vi "return zero.vi"(7 "Axis":enum16{"X", "Y", "X+Y"}(ring), 8 "error IN":errorcluster, 11 "Data IN":T1={"App State"="", "Connect "=FALSE, "phandle out"=0, "Axis"=[], "S ramp"=30.0, "Acceleration"=100000.0, "Initial Speed"=10.0, "Normal Open / Close"=enum."Close", "Deceleration"=100000.0, "Creep"=30.0, "Speed"=1000.0, "X Axis"={"Operating State"="", "Current Position"=0.0, "Current Speed"=0.0, "Axis State"=0, "Angle"=0.0}, "Y Axis"={"Operating State"="", "Current Position"=0.0, "Current Speed"=0.0, "Axis State"=0, "Angle"=0.0}, "Distance"=0.0, "Direct of movement"=enum."Forward", "Move Method"=enum."Continue", "Move Mode"=enum."Relative", "Angle"=enum."0", "Times"=0, "Start Time"=0.0, "Step Flag"=FALSE, "x  dist"=[], "y dist"=[], "x angle array"=[], "y angle array"=[], "index"=0.0, "big motion angle"=0.0, "big angle"=[], "xy dy speed table"=[], "x dy speed table"=[], "y dy speed table"=[], "x dy time"=[], "y dy time"=[], "xy dy time"=[], "dy Path  "=[]}) -> (0 "error out":errorcluster, 3 "Data out":T1={"App State"="", "Connect "=FALSE, "phandle out"=0, "Axis"=[], "S ramp"=30.0, "Acceleration"=100000.0, "Initial Speed"=10.0, "Normal Open / Close"=enum."Close", "Deceleration"=100000.0, "Creep"=30.0, "Speed"=1000.0, "X Axis"={"Operating State"="", "Current Position"=0.0, "Current Speed"=0.0, "Axis State"=0, "Angle"=0.0}, "Y Axis"={"Operating State"="", "Current Position"=0.0, "Current Speed"=0.0, "Axis State"=0, "Angle"=0.0}, "Distance"=0.0, "Direct of movement"=enum."Forward", "Move Method"=enum."Continue", "Move Mode"=enum."Relative", "Angle"=enum."0", "Times"=0, "Start Time"=0.0, "Step Flag"=FALSE, "x  dist"=[], "y dist"=[], "x angle array"=[], "y angle array"=[], "index"=0.0, "big motion angle"=0.0, "big angle"=[], "xy dy speed table"=[], "x dy speed table"=[], "y dy speed table"=[], "x dy time"=[], "y dy time"=[], "xy dy time"=[], "dy Path  "=[]})   [LabVIEW 2015]
uses:
  Typedef/Data2.ctl
  zauxdll-2014/zauxdll.lvlib
panel:
  # "m"
  # "m"
  # "m"
  # "m"
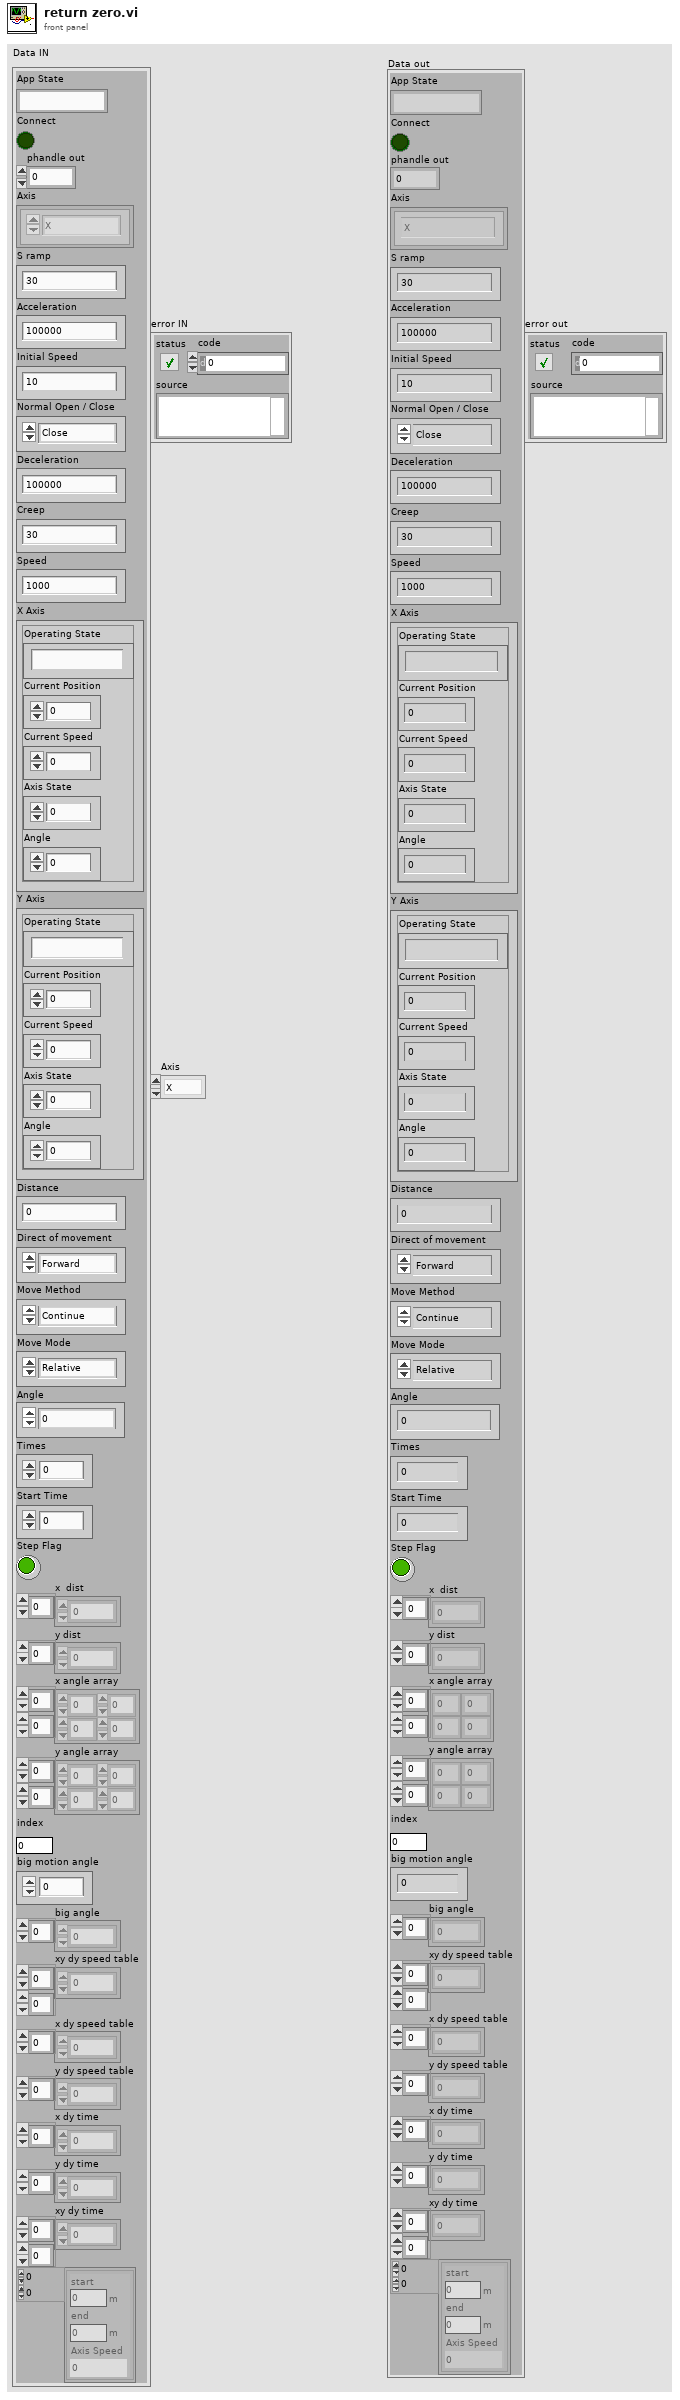
[diagram p1: front panel]
types:
  T1 = typedef "Data2.ctl" = cluster{"App State":string, "Connect ":bool, "phandle out":u32, "Axis":enum16{"X", "Y", "X+Y"}[], "S ramp":dbl, "Acceleration":dbl, "Initial Speed":dbl, "Normal Open / Close":enum16{"Open", "Close"}, "Deceleration":dbl, "Creep":dbl, "Speed":dbl, "X Axis":cluster{"Operating State":string, "Current Position":dbl, "Current Speed":dbl, "Axis State":i32, "Angle":dbl}, "Y Axis":cluster{"Operating State":string, "Current Position":dbl, "Current Speed":dbl, "Axis State":i32, "Angle":dbl}, "Distance":dbl, "Direct of movement":enum16{"Forward", "Backward"}, "Move Method":enum16{"Continue", "Inching"}, "Move Mode":enum16{"Relative", "Absolute"}, "Angle":enum32{"0", "1", "10", "30", "34", "60", "90", "180", "-1", "-10"}, "Times":i32, "Start Time":dbl, "Step Flag":bool, "x  dist":dbl[], "y dist":dbl[], "x angle array":i32[][], "y angle array":i32[][], "index":dbl, "big motion angle":dbl, "big angle":dbl[], "xy dy speed table":dbl[][], "x dy speed table":dbl[], "y dy speed table":dbl[], "x dy time":dbl[], "y dy time":dbl[], "xy dy time":dbl[][], "dy Path  ":cluster{"end":dbl, "start":dbl, "Axis Speed":dbl}[][]}
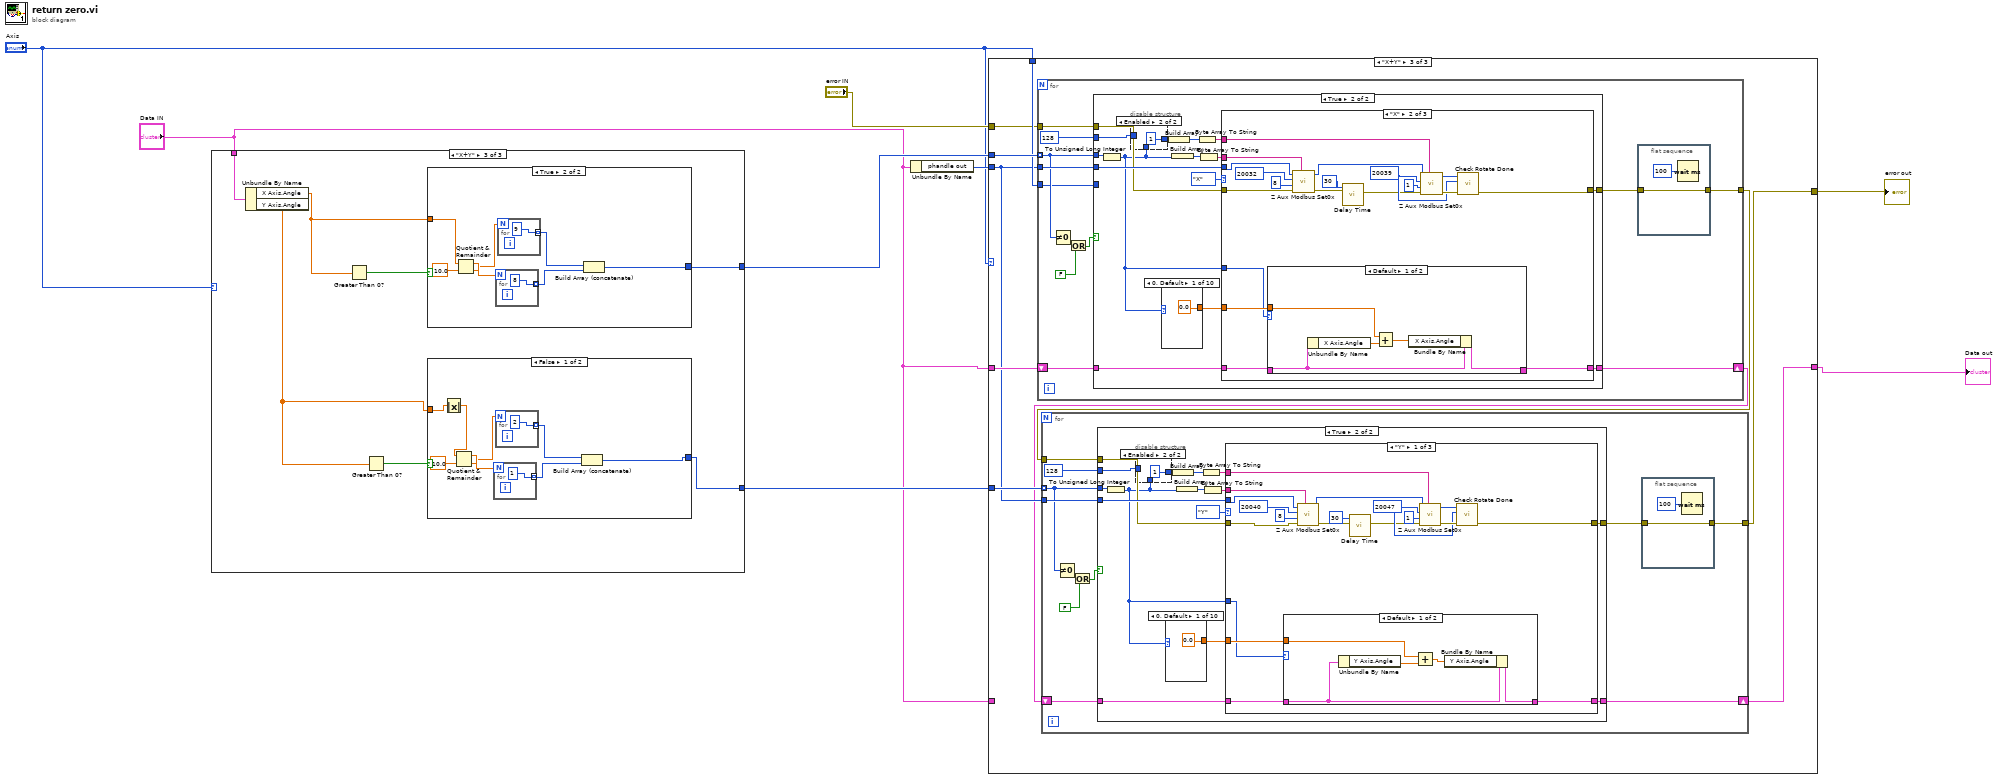
[diagram p0: block diagram]
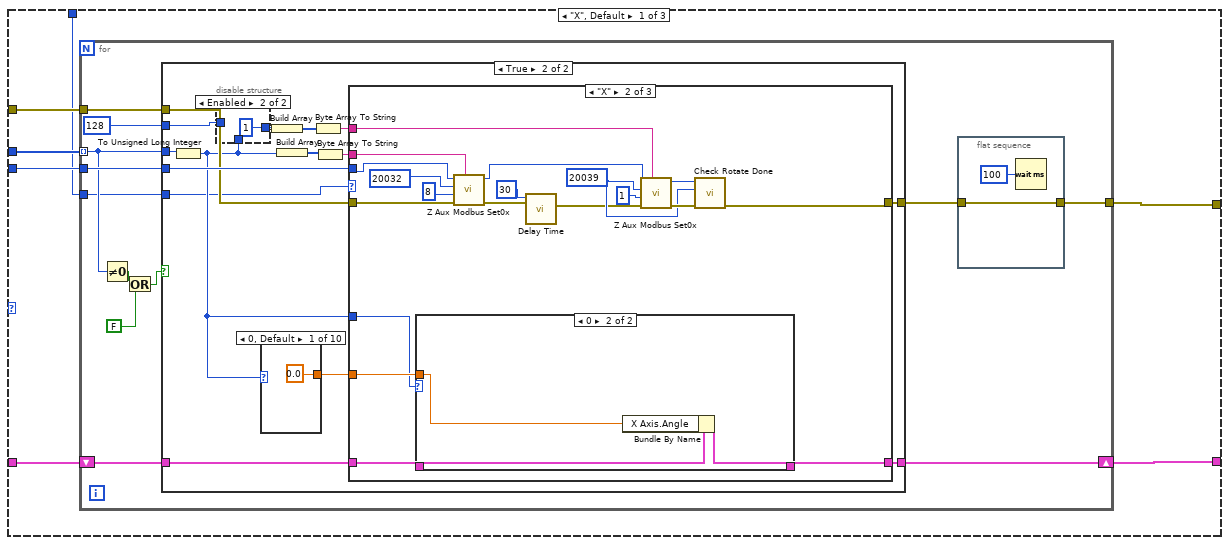
[diagram p2: hidden frame]
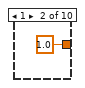
[diagram p4: hidden frame]
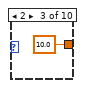
[diagram p5: hidden frame]
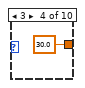
[diagram p6: hidden frame]
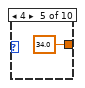
[diagram p7: hidden frame]
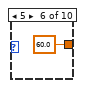
[diagram p8: hidden frame]
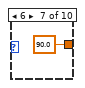
[diagram p9: hidden frame]
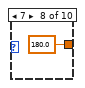
[diagram p10: hidden frame]
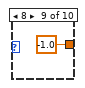
[diagram p11: hidden frame]
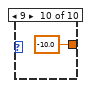
[diagram p12: hidden frame]
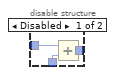
[diagram p13: hidden frame]
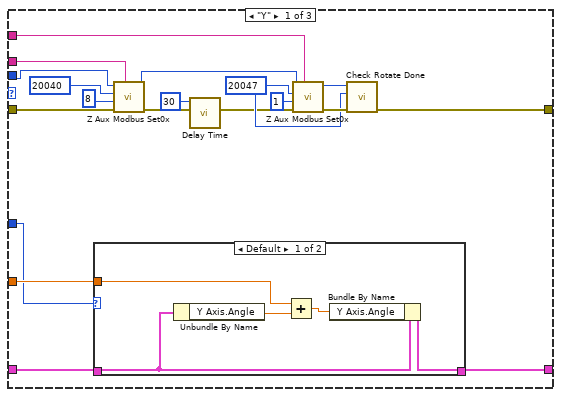
[diagram p14: hidden frame]
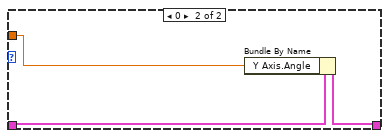
[diagram p15: hidden frame]
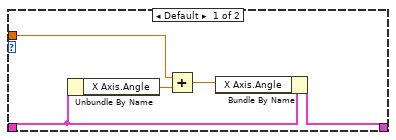
[diagram p16: hidden frame]
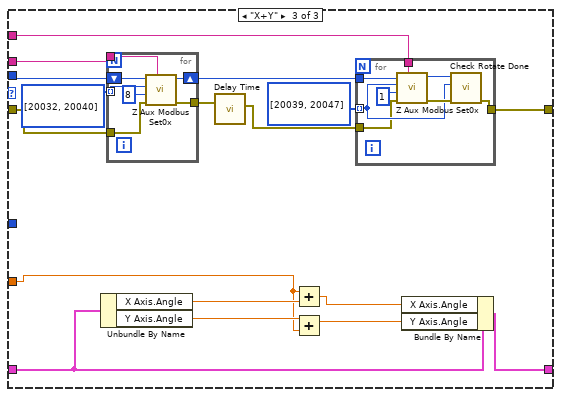
[diagram p17: hidden frame]
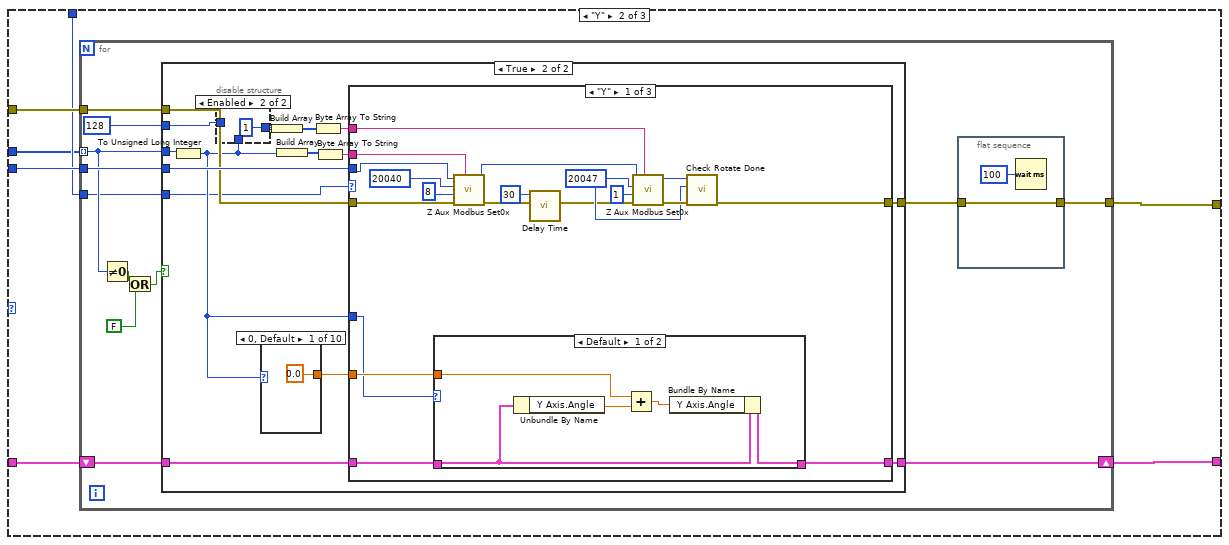
[diagram p18: hidden frame]
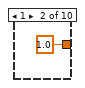
[diagram p20: hidden frame]
diagram:
  n1 = case shown="\"X+Y\"" "Axis" {
    tunnel: "Data IN" -> [w12 w35 w61]
    tunnel: [w9 w32 w58] -> w6
    tunnel: [_ _ w55] -> w4
    frame "X", Default {
      n2 = Unbundle By Name(w12) -> ("X Axis.Angle"=w10:dbl)
      n3 = Greater Than 0?(x=w10) -> (x > 0?=w11:bool)
      n4 = case shown="True" w11 {
        tunnel: w10 -> [w14 w29]
        tunnel: [w15 w23] -> w9
        frame False {
          n5 = Absolute Value(x=w14) -> (abs(x)=w13:dbl)
          n6 = Quotient & Remainder(x=w13, y=10.0) -> (x-y*floor(x/y)=w19:dbl, floor(x/y)=w18:dbl)
          n7 = for {
            N: w19 -> [_]
            tunnel: [1] -> w16 mode=indexing
          }
          n8 = for {
            N: w18 -> [_]
            tunnel: [2] -> w17 mode=indexing
          }
          n9 = Build Array (concatenate)(w17, w16) -> (w15:i32[])
        }
        frame True {
          n10 = Quotient & Remainder(x=w29, y=10.0) -> (x-y*floor(x/y)=w27:dbl, floor(x/y)=w26:dbl)
          n11 = for {
            N: w27 -> [_]
            tunnel: [8] -> w24 mode=indexing
          }
          n12 = for {
            N: w26 -> [_]
            tunnel: [9] -> w25 mode=indexing
          }
          n13 = Build Array (concatenate)(w25, w24) -> (w23:i32[])
        }
      }
    }
    frame "Y" {
      n14 = Unbundle By Name(w35) -> ("Y Axis.Angle"=w33:dbl)
      n15 = Greater Than 0?(x=w33) -> (x > 0?=w34:bool)
      n16 = case shown="True" w34 {
        tunnel: w33 -> [w37 w52]
        tunnel: [w38 w46] -> w32
        frame False {
          n17 = Absolute Value(x=w37) -> (abs(x)=w36:dbl)
          n18 = Quotient & Remainder(x=w36, y=10.0) -> (x-y*floor(x/y)=w42:dbl, floor(x/y)=w41:dbl)
          n19 = for {
            N: w42 -> [_]
            tunnel: [1] -> w39 mode=indexing
          }
          n20 = for {
            N: w41 -> [_]
            tunnel: [2] -> w40 mode=indexing
          }
          n21 = Build Array (concatenate)(w40, w39) -> (w38:i32[])
        }
        frame True {
          n22 = Quotient & Remainder(x=w52, y=10.0) -> (x-y*floor(x/y)=w50:dbl, floor(x/y)=w49:dbl)
          n23 = for {
            N: w50 -> [_]
            tunnel: [8] -> w47 mode=indexing
          }
          n24 = for {
            N: w49 -> [_]
            tunnel: [9] -> w48 mode=indexing
          }
          n25 = Build Array (concatenate)(w48, w47) -> (w46:i32[])
        }
      }
    }
    frame "X+Y" {
      n26 = Unbundle By Name(w61) -> ("X Axis.Angle"=w59:dbl, "Y Axis.Angle"=w56:dbl)
      n27 = Greater Than 0?(x=w59) -> (x > 0?=w60:bool)
      n28 = Greater Than 0?(x=w56) -> (x > 0?=w57:bool)
      n29 = case shown="True" w60 {
        tunnel: w59 -> [w82 w97]
        tunnel: [w83 w91] -> w58
        frame False {
          n30 = Absolute Value(x=w82) -> (abs(x)=w81:dbl)
          n31 = Quotient & Remainder(x=w81, y=10.0) -> (x-y*floor(x/y)=w87:dbl, floor(x/y)=w86:dbl)
          n32 = for {
            N: w87 -> [_]
            tunnel: [1] -> w84 mode=indexing
          }
          n33 = for {
            N: w86 -> [_]
            tunnel: [2] -> w85 mode=indexing
          }
          n34 = Build Array (concatenate)(w85, w84) -> (w83:i32[])
        }
        frame True {
          n35 = Quotient & Remainder(x=w97, y=10.0) -> (x-y*floor(x/y)=w95:dbl, floor(x/y)=w94:dbl)
          n36 = for {
            N: w95 -> [_]
            tunnel: [8] -> w92 mode=indexing
          }
          n37 = for {
            N: w94 -> [_]
            tunnel: [9] -> w93 mode=indexing
          }
          n38 = Build Array (concatenate)(w93, w92) -> (w91:i32[])
        }
      }
      n39 = case shown="False" w57 {
        tunnel: w56 -> [w63 w78]
        tunnel: [w64 w72] -> w55
        frame False {
          n40 = Absolute Value(x=w63) -> (abs(x)=w62:dbl)
          n41 = Quotient & Remainder(x=w62, y=10.0) -> (x-y*floor(x/y)=w68:dbl, floor(x/y)=w67:dbl)
          n42 = for {
            N: w68 -> [_]
            tunnel: [1] -> w65 mode=indexing
          }
          n43 = for {
            N: w67 -> [_]
            tunnel: [2] -> w66 mode=indexing
          }
          n44 = Build Array (concatenate)(w66, w65) -> (w64:i32[])
        }
        frame True {
          n45 = Quotient & Remainder(x=w78, y=10.0) -> (x-y*floor(x/y)=w76:dbl, floor(x/y)=w75:dbl)
          n46 = for {
            N: w76 -> [_]
            tunnel: [8] -> w73 mode=indexing
          }
          n47 = for {
            N: w75 -> [_]
            tunnel: [9] -> w74 mode=indexing
          }
          n48 = Build Array (concatenate)(w74, w73) -> (w72:i32[])
        }
      }
    }
  }
  n49 = Unbundle By Name("Data IN") -> ("phandle out"=w8:u32)
  n50 = case shown="\"X+Y\"" "Axis" {
    tunnel: w8 -> [w106 w244 w380]
    tunnel: "error IN" -> [w105 w243 w382]
    tunnel: "Data IN" -> [w104 w242 w385]
    tunnel: w6 -> [w103 w238 w384]
    tunnel: [w102 w241 w377] -> w1
    tunnel: "Axis" -> [w101 w240 w383]
    tunnel: w4 -> [_ _ w381]
    tunnel: "Data IN" -> [_ _ _]
    tunnel: [w100 w239 w378] -> w2
    frame "X", Default {
      n51 = for {
        tunnel: w106 -> [w114]
        tunnel: w105 -> [w118]
        tunnel: w103 -> [w113] mode=indexing
        shift-right: [w115] -> w102
        shift-left: w104 -> [w116]
        tunnel: [w109] -> w100
        tunnel: w101 -> [w107]
        n52 = Not Equal To 0?(x=w113) -> (x != 0?=w111:bool)
        n53 = Or(x=w111, y=FALSE) -> (x .or. y?=w112:bool)
        n54 = case shown="True" w112 {
          tunnel: w114 -> [_ w137]
          tunnel: w118 -> [w122 w136]
          tunnel: u32 128 -> [_ w135]
          tunnel: w116 -> [w121 w129]
          tunnel: w113 -> [_ w128]
          tunnel: [w121 w127] -> w115
          tunnel: [w122 w126] -> w110
          tunnel: w107 -> [_ w123]
          frame False {
          }
          frame True {
            n55 = To Unsigned Long Integer(number=w128) -> (unsigned 32bit integer=w124:u32)
            n56 = disable-structure shown="Enabled" {
              disable-tunnel: w135 -> [w150 _]
              disable-tunnel: [w149 u32 1] -> w134
              disable-tunnel: w124 -> [w148 _]
              frame Disabled {
                n57 = Add(x=w150, y=w148) -> (x+y=w149:u32)
              }
              frame Enabled {
              }
            }
            n58 = case shown="0, Default" w124 {
              tunnel: [0.0 1.0 10.0 30.0 34.0 60.0 90.0 180.0 -1.0 -10.0] -> w130
              frame 0, Default {
              }
              frame 1 {
              }
              frame 2 {
              }
              frame 3 {
              }
              frame 4 {
              }
              frame 5 {
              }
              frame 6 {
              }
              frame 7 {
              }
              frame 8 {
              }
              frame 9 {
              }
            }
            n59 = Build Array(w134) -> (w133:u32[])
            n60 = Build Array(w124) -> (w125:u32[])
            n61 = Byte Array To String(unsigned byte array=w133) -> (string=w132:string)
            n62 = Byte Array To String(unsigned byte array=w125) -> (string=w131:string)
            n63 = case shown="\"X\"" w123 {
              tunnel: w137 -> [w167 w194 w221]
              tunnel: w132 -> [w168 w195 w222]
              tunnel: w131 -> [w166 w193 w220]
              tunnel: w136 -> [w161 w188 w217]
              tunnel: [w156 w183 w213] -> w126
              tunnel: w129 -> [w155 w182 w210]
              tunnel: [w154 w181 w209] -> w127
              tunnel: w130 -> [w153 w180 w206]
              tunnel: w124 -> [w152 w179 _]
              frame "Y" {
                w162 = u16 20047 ("start")
                n64 = case shown="Default" w152 {
                  tunnel: w155 -> [w175 w178]
                  tunnel: [w174 w177] -> w154
                  tunnel: w153 -> [w171 w176]
                  frame Default {
                    n65 = Unbundle By Name(w175) -> ("Y Axis.Angle"=w172:dbl)
                    n66 = Add(x=w171, y=w172) -> (x+y=w173:dbl)
                    n67 = Bundle By Name(cluster=w175, "Y Axis.Angle"=w173) -> (w174:T1)
                  }
                  frame 0 {
                    n68 = Bundle By Name(cluster=w178, "Y Axis.Angle"=w176) -> (w177:T1)
                  }
                }
                n69 = call "Z Aux Modbus Set0x.vi"("pdata"=w166, "error in (no error)"=w161, "inum"=u16 8, "start"=u16 20040, "handle"=w167) -> ("error out"=w159:errorcluster, "handle out"=w160:u32)  [unwired: 3 in, 2 out]
                n70 = call "Delay Time.vi"("error in (no error)"=w159, "Delay(ms)"=u32 30) -> ("error out"=w157:errorcluster)  [unwired: 9 in]
                n71 = call "Z Aux Modbus Set0x.vi"("pdata"=w168, "error in (no error)"=w157, "inum"=u16 1, "start"=w162, "handle"=w160) -> ("error out"=w170:errorcluster, "handle out"=w169:u32)  [unwired: 3 in, 2 out]
                n72 = call "Check Rotate Done.vi"("error in (no error)"=w170, "start"=w162, "phandle in"=w169) -> ("error out"=w156:errorcluster)  [unwired: 8 in]
              }
              frame "X" {
                w189 = u16 20039 ("start")
                n73 = case shown="0" w179 {
                  tunnel: w182 -> [w202 w205]
                  tunnel: [w201 w204] -> w181
                  tunnel: w180 -> [w198 w203]
                  frame Default {
                    n74 = Unbundle By Name(w202) -> ("X Axis.Angle"=w200:dbl)
                    n75 = Add(x=w198, y=w200) -> (x+y=w199:dbl)
                    n76 = Bundle By Name(cluster=w202, "X Axis.Angle"=w199) -> (w201:T1)
                  }
                  frame 0 {
                    n77 = Bundle By Name(cluster=w205, "X Axis.Angle"=w203) -> (w204:T1)
                  }
                }
                n78 = call "Z Aux Modbus Set0x.vi"("pdata"=w193, "error in (no error)"=w188, "inum"=u16 8, "start"=u16 20032, "handle"=w194) -> ("error out"=w186:errorcluster, "handle out"=w187:u32)  [unwired: 3 in, 2 out]
                n79 = call "Delay Time.vi"("error in (no error)"=w186, "Delay(ms)"=u32 30) -> ("error out"=w184:errorcluster)  [unwired: 9 in]
                n80 = call "Z Aux Modbus Set0x.vi"("pdata"=w195, "error in (no error)"=w184, "inum"=u16 1, "start"=w189, "handle"=w187) -> ("error out"=w197:errorcluster, "handle out"=w196:u32)  [unwired: 3 in, 2 out]
                n81 = call "Check Rotate Done.vi"("error in (no error)"=w197, "start"=w189, "phandle in"=w196) -> ("error out"=w183:errorcluster)  [unwired: 8 in]
              }
              frame "X+Y" {
                n82 = Unbundle By Name(w210) -> ("X Axis.Angle"=w212:dbl, "Y Axis.Angle"=w211:dbl)
                n83 = for {
                  tunnel: w220 -> [w236]
                  shift-right: [w235] -> w215
                  shift-left: w221 -> [w237]
                  tunnel: i32[] [20032, 20040] -> [w233] mode=indexing
                  tunnel: w217 -> [w232]
                  tunnel: [w231] -> w216
                  n84 = call "Z Aux Modbus Set0x.vi"("pdata"=w236, "error in (no error)"=w232, "inum"=u16 8, "start"=w233, "handle"=w237) -> ("error out"=w231:errorcluster, "handle out"=w235:u32)  [unwired: 3 in, 2 out]
                }
                n85 = call "Delay Time.vi"("error in (no error)"=w216) -> ("error out"=w214:errorcluster)  [unwired: 10 in]
                n86 = Add(x=w206, y=w212) -> (x+y=w208:dbl)
                n87 = Add(x=w211, y=w206) -> (x+y=w207:dbl)
                n88 = for {
                  tunnel: w222 -> [w228]
                  tunnel: w215 -> [w227]
                  tunnel: i32[] [20039, 20047] -> [w225] mode=indexing
                  tunnel: w214 -> [w224]
                  tunnel: [w223] -> w213
                  n89 = call "Z Aux Modbus Set0x.vi"("pdata"=w228, "error in (no error)"=w224, "inum"=u16 1, "start"=w225, "handle"=w227) -> ("error out"=w230:errorcluster, "handle out"=w229:u32)  [unwired: 3 in, 2 out]
                  n90 = call "Check Rotate Done.vi"("error in (no error)"=w230, "start"=w225, "phandle in"=w229) -> ("error out"=w223:errorcluster)  [unwired: 8 in]
                }
                n91 = Bundle By Name(cluster=w210, "X Axis.Angle"=w208, "Y Axis.Angle"=w207) -> (w209:T1)
              }
            }
          }
        }
        n92 = flat-sequence {
          tunnel: w110 -> [w120]
          tunnel: [w120] -> w109
          frame #0 {
            n93 = Wait (ms)(milliseconds to wait=u32 100) -> ()  [unwired: 1 out]
          }
        }
      }
    }
    frame "Y" {
      n94 = for {
        tunnel: w244 -> [w252]
        tunnel: w243 -> [w256]
        tunnel: w238 -> [w251] mode=indexing
        shift-right: [w253] -> w241
        shift-left: w242 -> [w254]
        tunnel: [w247] -> w239
        tunnel: w240 -> [w245]
        n95 = Not Equal To 0?(x=w251) -> (x != 0?=w249:bool)
        n96 = Or(x=w249, y=FALSE) -> (x .or. y?=w250:bool)
        n97 = case shown="True" w250 {
          tunnel: w252 -> [_ w275]
          tunnel: w256 -> [w260 w274]
          tunnel: u32 128 -> [_ w273]
          tunnel: w254 -> [w259 w267]
          tunnel: w251 -> [_ w266]
          tunnel: [w259 w265] -> w253
          tunnel: [w260 w264] -> w248
          tunnel: w245 -> [_ w261]
          frame False {
          }
          frame True {
            n98 = To Unsigned Long Integer(number=w266) -> (unsigned 32bit integer=w262:u32)
            n99 = disable-structure shown="Enabled" {
              disable-tunnel: w273 -> [w288 _]
              disable-tunnel: [w287 u32 1] -> w272
              disable-tunnel: w262 -> [w286 _]
              frame Disabled {
                n100 = Add(x=w288, y=w286) -> (x+y=w287:u32)
              }
              frame Enabled {
              }
            }
            n101 = case shown="0, Default" w262 {
              tunnel: [0.0 1.0 10.0 30.0 34.0 60.0 90.0 180.0 -1.0 -10.0] -> w268
              frame 0, Default {
              }
              frame 1 {
              }
              frame 2 {
              }
              frame 3 {
              }
              frame 4 {
              }
              frame 5 {
              }
              frame 6 {
              }
              frame 7 {
              }
              frame 8 {
              }
              frame 9 {
              }
            }
            n102 = Build Array(w272) -> (w271:u32[])
            n103 = Build Array(w262) -> (w263:u32[])
            n104 = Byte Array To String(unsigned byte array=w271) -> (string=w270:string)
            n105 = Byte Array To String(unsigned byte array=w263) -> (string=w269:string)
            n106 = case shown="\"Y\"" w261 {
              tunnel: w275 -> [w305 w332 w359]
              tunnel: w270 -> [w306 w333 w360]
              tunnel: w269 -> [w304 w331 w358]
              tunnel: w274 -> [w299 w326 w355]
              tunnel: [w294 w321 w351] -> w264
              tunnel: w267 -> [w293 w320 w348]
              tunnel: [w292 w319 w347] -> w265
              tunnel: w268 -> [w291 w318 w344]
              tunnel: w262 -> [w290 w317 _]
              frame "Y" {
                w300 = u16 20047 ("start")
                n107 = case shown="Default" w290 {
                  tunnel: w293 -> [w313 w316]
                  tunnel: [w312 w315] -> w292
                  tunnel: w291 -> [w309 w314]
                  frame Default {
                    n108 = Unbundle By Name(w313) -> ("Y Axis.Angle"=w310:dbl)
                    n109 = Add(x=w309, y=w310) -> (x+y=w311:dbl)
                    n110 = Bundle By Name(cluster=w313, "Y Axis.Angle"=w311) -> (w312:T1)
                  }
                  frame 0 {
                    n111 = Bundle By Name(cluster=w316, "Y Axis.Angle"=w314) -> (w315:T1)
                  }
                }
                n112 = call "Z Aux Modbus Set0x.vi"("pdata"=w304, "error in (no error)"=w299, "inum"=u16 8, "start"=u16 20040, "handle"=w305) -> ("error out"=w297:errorcluster, "handle out"=w298:u32)  [unwired: 3 in, 2 out]
                n113 = call "Delay Time.vi"("error in (no error)"=w297, "Delay(ms)"=u32 30) -> ("error out"=w295:errorcluster)  [unwired: 9 in]
                n114 = call "Z Aux Modbus Set0x.vi"("pdata"=w306, "error in (no error)"=w295, "inum"=u16 1, "start"=w300, "handle"=w298) -> ("error out"=w308:errorcluster, "handle out"=w307:u32)  [unwired: 3 in, 2 out]
                n115 = call "Check Rotate Done.vi"("error in (no error)"=w308, "start"=w300, "phandle in"=w307) -> ("error out"=w294:errorcluster)  [unwired: 8 in]
              }
              frame "X" {
                w327 = u16 20039 ("start")
                n116 = case shown="0" w317 {
                  tunnel: w320 -> [w340 w343]
                  tunnel: [w339 w342] -> w319
                  tunnel: w318 -> [w336 w341]
                  frame Default {
                    n117 = Unbundle By Name(w340) -> ("X Axis.Angle"=w338:dbl)
                    n118 = Add(x=w336, y=w338) -> (x+y=w337:dbl)
                    n119 = Bundle By Name(cluster=w340, "X Axis.Angle"=w337) -> (w339:T1)
                  }
                  frame 0 {
                    n120 = Bundle By Name(cluster=w343, "X Axis.Angle"=w341) -> (w342:T1)
                  }
                }
                n121 = call "Z Aux Modbus Set0x.vi"("pdata"=w331, "error in (no error)"=w326, "inum"=u16 8, "start"=u16 20032, "handle"=w332) -> ("error out"=w324:errorcluster, "handle out"=w325:u32)  [unwired: 3 in, 2 out]
                n122 = call "Delay Time.vi"("error in (no error)"=w324, "Delay(ms)"=u32 30) -> ("error out"=w322:errorcluster)  [unwired: 9 in]
                n123 = call "Z Aux Modbus Set0x.vi"("pdata"=w333, "error in (no error)"=w322, "inum"=u16 1, "start"=w327, "handle"=w325) -> ("error out"=w335:errorcluster, "handle out"=w334:u32)  [unwired: 3 in, 2 out]
                n124 = call "Check Rotate Done.vi"("error in (no error)"=w335, "start"=w327, "phandle in"=w334) -> ("error out"=w321:errorcluster)  [unwired: 8 in]
              }
              frame "X+Y" {
                n125 = Unbundle By Name(w348) -> ("X Axis.Angle"=w350:dbl, "Y Axis.Angle"=w349:dbl)
                n126 = for {
                  tunnel: w358 -> [w374]
                  shift-right: [w373] -> w353
                  shift-left: w359 -> [w375]
                  tunnel: i32[] [20032, 20040] -> [w371] mode=indexing
                  tunnel: w355 -> [w370]
                  tunnel: [w369] -> w354
                  n127 = call "Z Aux Modbus Set0x.vi"("pdata"=w374, "error in (no error)"=w370, "inum"=u16 8, "start"=w371, "handle"=w375) -> ("error out"=w369:errorcluster, "handle out"=w373:u32)  [unwired: 3 in, 2 out]
                }
                n128 = call "Delay Time.vi"("error in (no error)"=w354) -> ("error out"=w352:errorcluster)  [unwired: 10 in]
                n129 = Add(x=w344, y=w350) -> (x+y=w346:dbl)
                n130 = Add(x=w349, y=w344) -> (x+y=w345:dbl)
                n131 = for {
                  tunnel: w360 -> [w366]
                  tunnel: w353 -> [w365]
                  tunnel: i32[] [20039, 20047] -> [w363] mode=indexing
                  tunnel: w352 -> [w362]
                  tunnel: [w361] -> w351
                  n132 = call "Z Aux Modbus Set0x.vi"("pdata"=w366, "error in (no error)"=w362, "inum"=u16 1, "start"=w363, "handle"=w365) -> ("error out"=w368:errorcluster, "handle out"=w367:u32)  [unwired: 3 in, 2 out]
                  n133 = call "Check Rotate Done.vi"("error in (no error)"=w368, "start"=w363, "phandle in"=w367) -> ("error out"=w361:errorcluster)  [unwired: 8 in]
                }
                n134 = Bundle By Name(cluster=w348, "X Axis.Angle"=w346, "Y Axis.Angle"=w345) -> (w347:T1)
              }
            }
          }
        }
        n135 = flat-sequence {
          tunnel: w248 -> [w258]
          tunnel: [w258] -> w247
          frame #0 {
            n136 = Wait (ms)(milliseconds to wait=u32 100) -> ()  [unwired: 1 out]
          }
        }
      }
    }
    frame "X+Y" {
      n137 = for {
        tunnel: w380 -> [w523]
        tunnel: w382 -> [w527]
        tunnel: w384 -> [w522] mode=indexing
        shift-right: [w524] -> w376
        shift-left: w385 -> [w525]
        tunnel: [w516] -> w379
        tunnel: w383 -> [w517]
        n138 = Not Equal To 0?(x=w522) -> (x != 0?=w520:bool)
        n139 = Or(x=w520, y=FALSE) -> (x .or. y?=w521:bool)
        n140 = case shown="True" w521 {
          tunnel: w523 -> [_ w546]
          tunnel: w527 -> [w531 w545]
          tunnel: u32 128 -> [_ w544]
          tunnel: w525 -> [w530 w538]
          tunnel: w522 -> [_ w537]
          tunnel: [w530 w536] -> w524
          tunnel: [w531 w535] -> w519
          tunnel: w517 -> [_ _]
          frame False {
          }
          frame True {
            n141 = To Unsigned Long Integer(number=w537) -> (unsigned 32bit integer=w533:u32)
            n142 = disable-structure shown="Enabled" {
              disable-tunnel: w544 -> [w559 _]
              disable-tunnel: [w558 u32 1] -> w543
              disable-tunnel: w533 -> [w557 _]
              frame Disabled {
                n143 = Add(x=w559, y=w557) -> (x+y=w558:u32)
              }
              frame Enabled {
              }
            }
            n144 = case shown="0, Default" w533 {
              tunnel: [0.0 1.0 10.0 30.0 34.0 60.0 90.0 180.0 -1.0 -10.0] -> w539
              frame 0, Default {
              }
              frame 1 {
              }
              frame 2 {
              }
              frame 3 {
              }
              frame 4 {
              }
              frame 5 {
              }
              frame 6 {
              }
              frame 7 {
              }
              frame 8 {
              }
              frame 9 {
              }
            }
            n145 = Build Array(w543) -> (w542:u32[])
            n146 = Build Array(w533) -> (w534:u32[])
            n147 = Byte Array To String(unsigned byte array=w542) -> (string=w541:string)
            n148 = Byte Array To String(unsigned byte array=w534) -> (string=w540:string)
            n149 = case shown="\"X\"" enum16{"X", "Y", "X+Y"}."X" ("Axis") {
              tunnel: w546 -> [w576 w603 w630]
              tunnel: w541 -> [w577 w604 w631]
              tunnel: w540 -> [w575 w602 w629]
              tunnel: w545 -> [w570 w597 w626]
              tunnel: [w565 w592 w622] -> w535
              tunnel: w538 -> [w564 w591 w619]
              tunnel: [w563 w590 w618] -> w536
              tunnel: w539 -> [w562 w589 w615]
              tunnel: w533 -> [w561 w588 _]
              frame "Y" {
                w571 = u16 20047 ("start")
                n150 = case shown="0" w561 {
                  tunnel: w564 -> [w584 w587]
                  tunnel: [w583 w586] -> w563
                  tunnel: w562 -> [w580 w585]
                  frame Default {
                    n151 = Unbundle By Name(w584) -> ("X Axis.Angle"=w581:dbl)
                    n152 = Add(x=w580, y=w581) -> (x+y=w582:dbl)
                    n153 = Bundle By Name(cluster=w584, "X Axis.Angle"=w582) -> (w583:T1)
                  }
                  frame 0 {
                    n154 = Bundle By Name(cluster=w587, "X Axis.Angle"=w585) -> (w586:T1)
                  }
                }
                n155 = call "Z Aux Modbus Set0x.vi"("pdata"=w575, "error in (no error)"=w570, "inum"=u16 8, "start"=u16 20040, "handle"=w576) -> ("error out"=w568:errorcluster, "handle out"=w569:u32)  [unwired: 3 in, 2 out]
                n156 = call "Delay Time.vi"("error in (no error)"=w568, "Delay(ms)"=u32 30) -> ("error out"=w566:errorcluster)  [unwired: 9 in]
                n157 = call "Z Aux Modbus Set0x.vi"("pdata"=w577, "error in (no error)"=w566, "inum"=u16 1, "start"=w571, "handle"=w569) -> ("error out"=w579:errorcluster, "handle out"=w578:u32)  [unwired: 3 in, 2 out]
                n158 = call "Check Rotate Done.vi"("error in (no error)"=w579, "start"=w571, "phandle in"=w578) -> ("error out"=w565:errorcluster)  [unwired: 8 in]
              }
              frame "X" {
                w598 = u16 20039 ("start")
                n159 = case shown="Default" w588 {
                  tunnel: w591 -> [w611 w614]
                  tunnel: [w610 w613] -> w590
                  tunnel: w589 -> [w607 w612]
                  frame Default {
                    n160 = Unbundle By Name(w611) -> ("X Axis.Angle"=w609:dbl)
                    n161 = Add(x=w607, y=w609) -> (x+y=w608:dbl)
                    n162 = Bundle By Name(cluster=w611, "X Axis.Angle"=w608) -> (w610:T1)
                  }
                  frame 0 {
                    n163 = Bundle By Name(cluster=w614, "X Axis.Angle"=w612) -> (w613:T1)
                  }
                }
                n164 = call "Z Aux Modbus Set0x.vi"("pdata"=w602, "error in (no error)"=w597, "inum"=u16 8, "start"=u16 20032, "handle"=w603) -> ("error out"=w595:errorcluster, "handle out"=w596:u32)  [unwired: 3 in, 2 out]
                n165 = call "Delay Time.vi"("error in (no error)"=w595, "Delay(ms)"=u32 30) -> ("error out"=w593:errorcluster)  [unwired: 9 in]
                n166 = call "Z Aux Modbus Set0x.vi"("pdata"=w604, "error in (no error)"=w593, "inum"=u16 1, "start"=w598, "handle"=w596) -> ("error out"=w606:errorcluster, "handle out"=w605:u32)  [unwired: 3 in, 2 out]
                n167 = call "Check Rotate Done.vi"("error in (no error)"=w606, "start"=w598, "phandle in"=w605) -> ("error out"=w592:errorcluster)  [unwired: 8 in]
              }
              frame "X+Y" {
                n168 = Unbundle By Name(w619) -> ("X Axis.Angle"=w621:dbl, "Y Axis.Angle"=w620:dbl)
                n169 = for {
                  tunnel: w629 -> [w645]
                  shift-right: [w644] -> w624
                  shift-left: w630 -> [w646]
                  tunnel: i32[] [20032, 20040] -> [w642] mode=indexing
                  tunnel: w626 -> [w641]
                  tunnel: [w640] -> w625
                  n170 = call "Z Aux Modbus Set0x.vi"("pdata"=w645, "error in (no error)"=w641, "inum"=u16 8, "start"=w642, "handle"=w646) -> ("error out"=w640:errorcluster, "handle out"=w644:u32)  [unwired: 3 in, 2 out]
                }
                n171 = call "Delay Time.vi"("error in (no error)"=w625) -> ("error out"=w623:errorcluster)  [unwired: 10 in]
                n172 = Add(x=w615, y=w621) -> (x+y=w617:dbl)
                n173 = Add(x=w620, y=w615) -> (x+y=w616:dbl)
                n174 = for {
                  tunnel: w631 -> [w637]
                  tunnel: w624 -> [w636]
                  tunnel: i32[] [20039, 20047] -> [w634] mode=indexing
                  tunnel: w623 -> [w633]
                  tunnel: [w632] -> w622
                  n175 = call "Z Aux Modbus Set0x.vi"("pdata"=w637, "error in (no error)"=w633, "inum"=u16 1, "start"=w634, "handle"=w636) -> ("error out"=w639:errorcluster, "handle out"=w638:u32)  [unwired: 3 in, 2 out]
                  n176 = call "Check Rotate Done.vi"("error in (no error)"=w639, "start"=w634, "phandle in"=w638) -> ("error out"=w632:errorcluster)  [unwired: 8 in]
                }
                n177 = Bundle By Name(cluster=w619, "X Axis.Angle"=w617, "Y Axis.Angle"=w616) -> (w618:T1)
              }
            }
          }
        }
        n178 = flat-sequence {
          tunnel: w519 -> [w529]
          tunnel: [w529] -> w516
          frame #0 {
            n179 = Wait (ms)(milliseconds to wait=u32 100) -> ()  [unwired: 1 out]
          }
        }
      }
      n180 = for {
        tunnel: w380 -> [w392]
        tunnel: w379 -> [w396]
        tunnel: w381 -> [w391] mode=indexing
        shift-right: [w393] -> w377
        shift-left: w376 -> [w394]
        tunnel: [w387] -> w378
        n181 = Not Equal To 0?(x=w391) -> (x != 0?=w389:bool)
        n182 = Or(x=w389, y=FALSE) -> (x .or. y?=w390:bool)
        n183 = case shown="True" w390 {
          tunnel: w392 -> [_ w415]
          tunnel: w396 -> [w400 w414]
          tunnel: u32 128 -> [_ w413]
          tunnel: w394 -> [w399 w407]
          tunnel: w391 -> [_ w406]
          tunnel: [w399 w405] -> w393
          tunnel: [w400 w404] -> w388
          frame False {
          }
          frame True {
            n184 = To Unsigned Long Integer(number=w406) -> (unsigned 32bit integer=w402:u32)
            n185 = disable-structure shown="Enabled" {
              disable-tunnel: w413 -> [w428 _]
              disable-tunnel: [w427 u32 1] -> w412
              disable-tunnel: w402 -> [w426 _]
              frame Disabled {
                n186 = Add(x=w428, y=w426) -> (x+y=w427:u32)
              }
              frame Enabled {
              }
            }
            n187 = case shown="0, Default" w402 {
              tunnel: [0.0 1.0 10.0 30.0 34.0 60.0 90.0 180.0 -1.0 -10.0] -> w408
              frame 0, Default {
              }
              frame 1 {
              }
              frame 2 {
              }
              frame 3 {
              }
              frame 4 {
              }
              frame 5 {
              }
              frame 6 {
              }
              frame 7 {
              }
              frame 8 {
              }
              frame 9 {
              }
            }
            n188 = Build Array(w412) -> (w411:u32[])
            n189 = Build Array(w402) -> (w403:u32[])
            n190 = Byte Array To String(unsigned byte array=w411) -> (string=w410:string)
            n191 = Byte Array To String(unsigned byte array=w403) -> (string=w409:string)
            n192 = case shown="\"Y\"" enum16{"X", "Y", "X+Y"}."Y" ("Axis") {
              tunnel: w415 -> [w445 w472 w499]
              tunnel: w410 -> [w446 w473 w500]
              tunnel: w409 -> [w444 w471 w498]
              tunnel: w414 -> [w430 w466 w495]
              tunnel: [w435 w461 w491] -> w404
              tunnel: w407 -> [w434 w460 w488]
              tunnel: [w433 w459 w487] -> w405
              tunnel: w408 -> [w432 w458 w484]
              tunnel: w402 -> [w431 w457 _]
              frame "Y" {
                w440 = u16 20047 ("start")
                n193 = case shown="Default" w431 {
                  tunnel: w434 -> [w453 w456]
                  tunnel: [w452 w455] -> w433
                  tunnel: w432 -> [w449 w454]
                  frame Default {
                    n194 = Unbundle By Name(w453) -> ("Y Axis.Angle"=w450:dbl)
                    n195 = Add(x=w449, y=w450) -> (x+y=w451:dbl)
                    n196 = Bundle By Name(cluster=w453, "Y Axis.Angle"=w451) -> (w452:T1)
                  }
                  frame 0 {
                    n197 = Bundle By Name(cluster=w456, "Y Axis.Angle"=w454) -> (w455:T1)
                  }
                }
                n198 = call "Z Aux Modbus Set0x.vi"("pdata"=w444, "error in (no error)"=w430, "inum"=u16 8, "start"=u16 20040, "handle"=w445) -> ("error out"=w438:errorcluster, "handle out"=w439:u32)  [unwired: 3 in, 2 out]
                n199 = call "Delay Time.vi"("error in (no error)"=w438, "Delay(ms)"=u32 30) -> ("error out"=w436:errorcluster)  [unwired: 9 in]
                n200 = call "Z Aux Modbus Set0x.vi"("pdata"=w446, "error in (no error)"=w436, "inum"=u16 1, "start"=w440, "handle"=w439) -> ("error out"=w448:errorcluster, "handle out"=w447:u32)  [unwired: 3 in, 2 out]
                n201 = call "Check Rotate Done.vi"("error in (no error)"=w448, "start"=w440, "phandle in"=w447) -> ("error out"=w435:errorcluster)  [unwired: 8 in]
              }
              frame "X" {
                w467 = u16 20039 ("start")
                n202 = case shown="0" w457 {
                  tunnel: w460 -> [w480 w483]
                  tunnel: [w479 w482] -> w459
                  tunnel: w458 -> [w476 w481]
                  frame Default {
                    n203 = Unbundle By Name(w480) -> ("X Axis.Angle"=w478:dbl)
                    n204 = Add(x=w476, y=w478) -> (x+y=w477:dbl)
                    n205 = Bundle By Name(cluster=w480, "X Axis.Angle"=w477) -> (w479:T1)
                  }
                  frame 0 {
                    n206 = Bundle By Name(cluster=w483, "X Axis.Angle"=w481) -> (w482:T1)
                  }
                }
                n207 = call "Z Aux Modbus Set0x.vi"("pdata"=w471, "error in (no error)"=w466, "inum"=u16 8, "start"=u16 20032, "handle"=w472) -> ("error out"=w464:errorcluster, "handle out"=w465:u32)  [unwired: 3 in, 2 out]
                n208 = call "Delay Time.vi"("error in (no error)"=w464, "Delay(ms)"=u32 30) -> ("error out"=w462:errorcluster)  [unwired: 9 in]
                n209 = call "Z Aux Modbus Set0x.vi"("pdata"=w473, "error in (no error)"=w462, "inum"=u16 1, "start"=w467, "handle"=w465) -> ("error out"=w475:errorcluster, "handle out"=w474:u32)  [unwired: 3 in, 2 out]
                n210 = call "Check Rotate Done.vi"("error in (no error)"=w475, "start"=w467, "phandle in"=w474) -> ("error out"=w461:errorcluster)  [unwired: 8 in]
              }
              frame "X+Y" {
                n211 = Unbundle By Name(w488) -> ("X Axis.Angle"=w490:dbl, "Y Axis.Angle"=w489:dbl)
                n212 = for {
                  tunnel: w498 -> [w514]
                  shift-right: [w513] -> w493
                  shift-left: w499 -> [w515]
                  tunnel: i32[] [20032, 20040] -> [w511] mode=indexing
                  tunnel: w495 -> [w510]
                  tunnel: [w509] -> w494
                  n213 = call "Z Aux Modbus Set0x.vi"("pdata"=w514, "error in (no error)"=w510, "inum"=u16 8, "start"=w511, "handle"=w515) -> ("error out"=w509:errorcluster, "handle out"=w513:u32)  [unwired: 3 in, 2 out]
                }
                n214 = call "Delay Time.vi"("error in (no error)"=w494) -> ("error out"=w492:errorcluster)  [unwired: 10 in]
                n215 = Add(x=w484, y=w490) -> (x+y=w486:dbl)
                n216 = Add(x=w489, y=w484) -> (x+y=w485:dbl)
                n217 = for {
                  tunnel: w500 -> [w506]
                  tunnel: w493 -> [w505]
                  tunnel: i32[] [20039, 20047] -> [w503] mode=indexing
                  tunnel: w492 -> [w502]
                  tunnel: [w501] -> w491
                  n218 = call "Z Aux Modbus Set0x.vi"("pdata"=w506, "error in (no error)"=w502, "inum"=u16 1, "start"=w503, "handle"=w505) -> ("error out"=w508:errorcluster, "handle out"=w507:u32)  [unwired: 3 in, 2 out]
                  n219 = call "Check Rotate Done.vi"("error in (no error)"=w508, "start"=w503, "phandle in"=w507) -> ("error out"=w501:errorcluster)  [unwired: 8 in]
                }
                n220 = Bundle By Name(cluster=w488, "X Axis.Angle"=w486, "Y Axis.Angle"=w485) -> (w487:T1)
              }
            }
          }
        }
        n221 = flat-sequence {
          tunnel: w388 -> [w398]
          tunnel: [w398] -> w387
          frame #0 {
            n222 = Wait (ms)(milliseconds to wait=u32 100) -> ()  [unwired: 1 out]
          }
        }
      }
    }
  }
  "Data out" <- w1
  "error out" <- w2
